vi "RD_StepMotor_WP.vi"(8 "Step resolution":u16(ring) items=["Full step", "Half step", "1/4 step", "1/8 step", "1/16 step", "1/32 step"], 9 "Direction":bool, 10 "Time between steps (ms)":i32=1, 11 "Steps":i64=1) -> ()   [LabVIEW 2014]
doc: "Random Laser Project\nAndré Romero - 2020\nandretec@ifsc.usp.br\n\nStep motor Control"
panel:
  out "Decimal number":u32
  # "DRV8825 Stepper Motor"
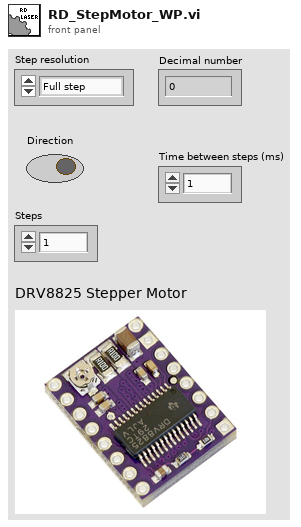
[diagram p1: front panel]
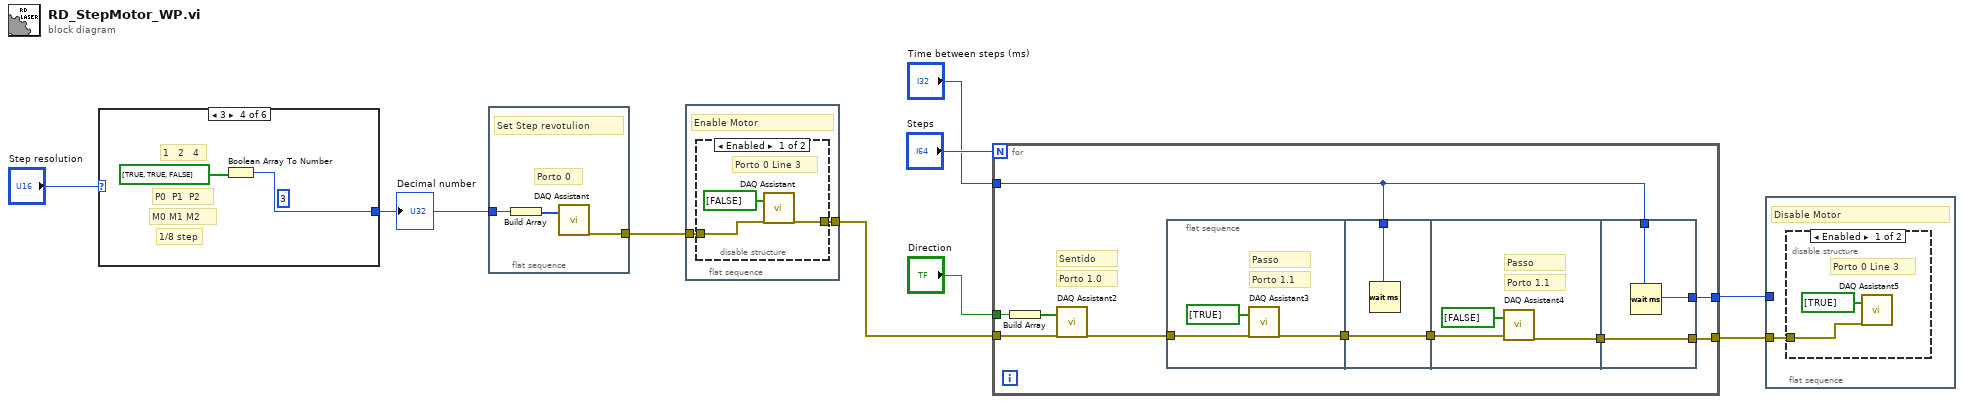
[diagram p0: block diagram]
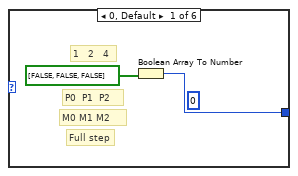
[diagram p4: hidden frame]
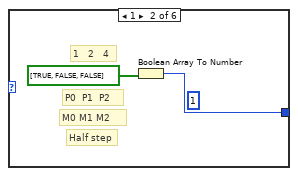
[diagram p5: hidden frame]
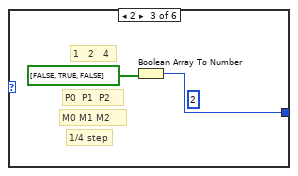
[diagram p6: hidden frame]
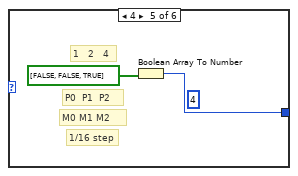
[diagram p7: hidden frame]
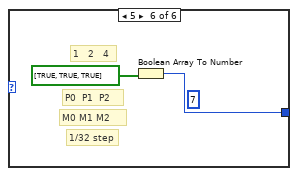
[diagram p8: hidden frame]
diagram:
  n1 = case shown="3" "Step resolution" {
    tunnel: [w10 w12 w14 w16 w18 w20] -> w9
    frame 0, Default {
      (unwired) 0
      # "Full step"
      # "M0 M1 M2"
      # "P0  P1  P2"
      # "1   2   4"
      n2 = Boolean Array To Number(Boolean array=bool[] [FALSE, FALSE, FALSE]) -> (number=w10:u32)
    }
    frame 1 {
      (unwired) 1
      # "Half step"
      # "M0 M1 M2"
      # "P0  P1  P2"
      # "1   2   4"
      n3 = Boolean Array To Number(Boolean array=bool[] [TRUE, FALSE, FALSE]) -> (number=w12:u32)
    }
    frame 2 {
      (unwired) 2
      # "1/4 step"
      # "M0 M1 M2"
      # "P0  P1  P2"
      # "1   2   4"
      n4 = Boolean Array To Number(Boolean array=bool[] [FALSE, TRUE, FALSE]) -> (number=w14:u32)
    }
    frame 3 {
      (unwired) 3
      # "1/8 step"
      # "M0 M1 M2"
      # "P0  P1  P2"
      # "1   2   4"
      n5 = Boolean Array To Number(Boolean array=bool[] [TRUE, TRUE, FALSE]) -> (number=w16:u32)
    }
    frame 4 {
      (unwired) 4
      # "1/16 step"
      # "M0 M1 M2"
      # "P0  P1  P2"
      # "1   2   4"
      n6 = Boolean Array To Number(Boolean array=bool[] [FALSE, FALSE, TRUE]) -> (number=w18:u32)
    }
    frame 5 {
      (unwired) 7
      # "1/32 step"
      # "M0 M1 M2"
      # "P0  P1  P2"
      # "1   2   4"
      n7 = Boolean Array To Number(Boolean array=bool[] [TRUE, TRUE, TRUE]) -> (number=w20:u32)
    }
  }
  "Decimal number" <- w9
  n8 = flat-sequence {
    tunnel: w9 -> [w23]
    tunnel: [w22] -> w3
    frame #0 {
      # "Porto 0"
      # "Set Step revotulion"
      n9 = Build Array(w23) -> (w24:u32[])
      n10 = call "DAQ Assistant"("data"=w24) -> ("error out"=w22:errorcluster)  [unwired: 17 in, 1 out]
    }
  }
  n11 = flat-sequence {
    tunnel: w3 -> [w26]
    tunnel: [w25] -> w2
    frame #0 {
      # "Enable Motor"
      n12 = disable-structure shown="Enabled" {
        disable-tunnel: w26 -> [w28 w30]
        disable-tunnel: [w27 w30] -> w25
        frame Enabled {
          # "Porto 0 Line 3"
          n13 = call "DAQ Assistant"("data"=bool[] [FALSE], "error in"=w28) -> ("error out"=w27:errorcluster)  [unwired: 16 in, 1 out]
        }
        frame Disabled {
        }
      }
    }
  }
  n14 = for {
    N: "Steps" -> [_]
    tunnel: "Direction" -> [w39]
    tunnel: "Time between steps (ms)" -> [w37]
    tunnel: [w34] -> w4
    tunnel: w2 -> [w33]
    tunnel: [w32] -> w1
    # "Sentido"
    # "Porto 1.0"
    n15 = Build Array(w39) -> (w40:bool[])
    n16 = call "DAQ Assistant2"("data"=w40, "error in"=w33) -> ("error out"=w38:errorcluster)  [unwired: 16 in, 1 out]
    n17 = flat-sequence {
      tunnel: w38 -> [w43]
      tunnel: [w41] -> w36
      tunnel: w37 -> [w45]
      tunnel: w36 -> [w44]
      tunnel: [w44] -> w35
      tunnel: w35 -> [w47]
      tunnel: [w46] -> w31
      tunnel: w37 -> [w50]
      tunnel: [w50] -> w34
      tunnel: [w49] -> w32
      tunnel: w31 -> [w49]
      frame #0 {
        # "Passo"
        # "Porto 1.1"
        n18 = call "DAQ Assistant3"("data"=bool[] [TRUE], "error in"=w43) -> ("error out"=w41:errorcluster)  [unwired: 16 in, 1 out]
      }
      frame #1 {
        n19 = Wait (ms)(milliseconds to wait=w45) -> ()  [unwired: 1 out]
      }
      frame #2 {
        # "Passo"
        # "Porto 1.1"
        n20 = call "DAQ Assistant4"("data"=bool[] [FALSE], "error in"=w47) -> ("error out"=w46:errorcluster)  [unwired: 16 in, 1 out]
      }
      frame #3 {
        n21 = Wait (ms)(milliseconds to wait=w50) -> ()  [unwired: 1 out]
      }
    }
  }
  n22 = flat-sequence {
    tunnel: w4 -> [_]
    tunnel: w1 -> [w51]
    frame #0 {
      # "Disable Motor"
      n23 = disable-structure shown="Enabled" {
        disable-tunnel: w51 -> [w52 _]
        frame Enabled {
          # "Porto 0 Line 3"
          n24 = call "DAQ Assistant5"("data"=bool[] [TRUE], "error in"=w52) -> ()  [unwired: 16 in, 2 out]
        }
        frame Disabled {
        }
      }
    }
  }
